vi "Entry.vi"(8 "error in (no error)":errorcluster, 11 "New State":refnum<class "Annoucing.lvclass">) -> (0 "error out":errorcluster, 3 "State out":refnum<class "Annoucing.lvclass">)   [LabVIEW 2013, in "Receiver.lvlib" / "Receive Commands Using State Actors.lvlib" / "Connect Command.lvlib" / "Executing States.lvlib" / "Annoucing.lvclass"]
doc: "This is an abstract method. Override this method to define the behavior when you enter the state."
uses:
  Annoucing.lvclass
  Executing State.lvclass
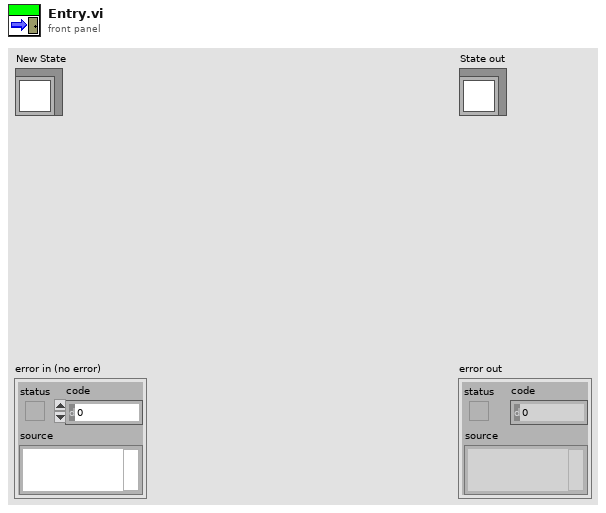
[diagram p1: front panel]
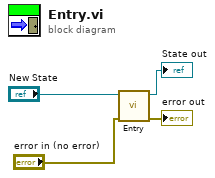
[diagram p0: block diagram]
diagram:
  n1 = call-parent "Entry.vi"("error in (no error)"="error in (no error)", "New State"="New State") -> ("error out"=→"error out":errorcluster, "State out"=→"State out":refnum<class "Annoucing.lvclass">)  [unwired: 8 in]
